vi "Write Name.vi"(8 "error in (no error)":errorcluster, 10 "Name":string, 11 "Process Generator In":refnum<class "Process Generator.lvclass">) -> (0 "error out":errorcluster, 3 "Process Generator Out":refnum<class "Process Generator.lvclass">)   [LabVIEW 2020, in "Process Generator.lvclass"]
uses:
  Process Generator.lvclass
  Process Generator.lvclass/Process Generator.ctl
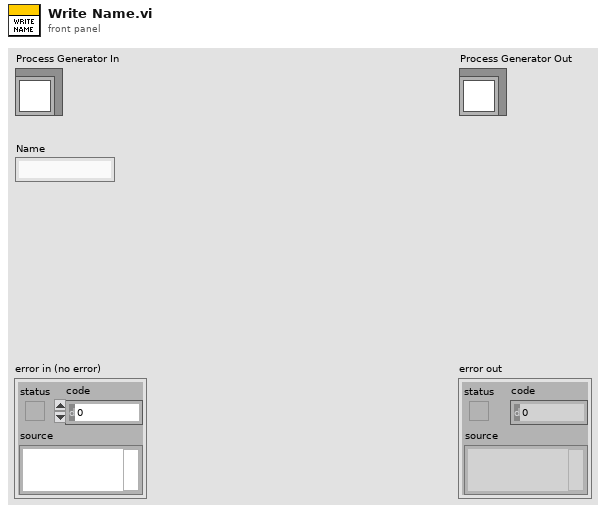
[diagram p1: front panel]
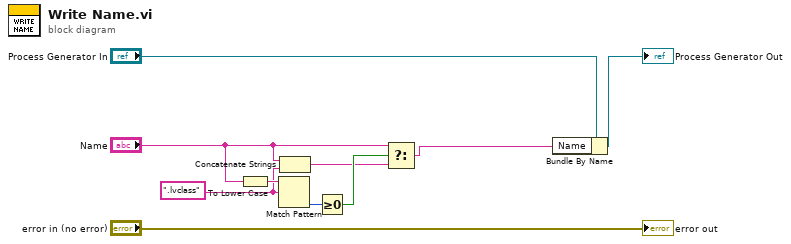
[diagram p0: block diagram]
diagram:
  w3 = ".lvclass"
  n1 = To Lower Case(string="Name") -> (all lower case string=w7:string)
  n2 = Match Pattern(string=w7, regular expression=w3) -> (offset past match=w6:i32)  [unwired: 1 in, 3 out]
  n3 = Concatenate Strings("Name", w3) -> (w1:string)
  n4 = Greater Or Equal To 0?(x=w6) -> (x >= 0?=w5:bool)
  n5 = Select(t="Name", s=w5, f=w1) -> (s? t:f=w4:string)
  n6 = Bundle By Name(cluster="Process Generator In", "Name"=w4) -> (→"Process Generator Out":refnum<class "Process Generator.lvclass">)
  "error out" <- "error in (no error)"
